vi "DAQ - close all tasks.vi"(8 "Frame Rate":refnum<k21>, 9 "Camera Gate":refnum<k21>, 10 "LED Gate":refnum<k21>, 11 "clock":refnum<k21>) -> (0 "error out":errorcluster)   [LabVIEW 2010]
panel:
  in  "error in":errorcluster
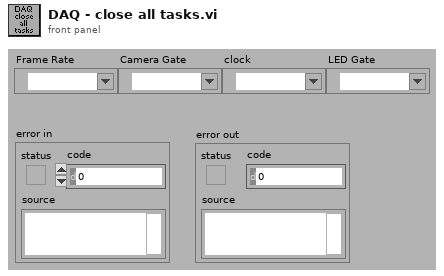
[diagram p1: front panel]
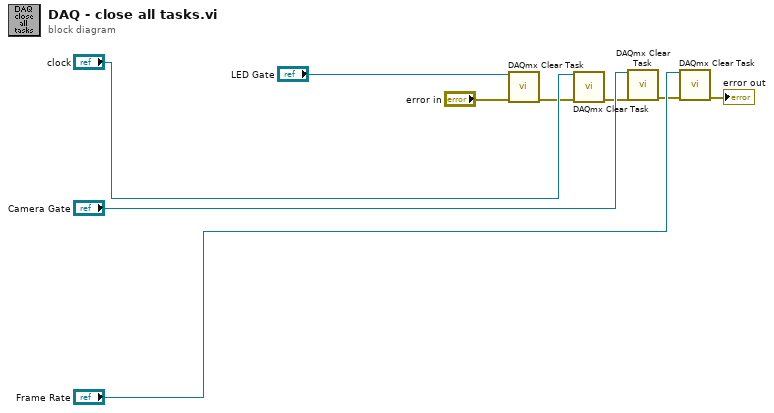
[diagram p0: block diagram]
diagram:
  n1 = call <vilib>:"DAQmx Clear Task.vi"("task in"="LED Gate", "error in"="error in") -> ("error out"=w4:errorcluster)  [unwired: 13 in]
  n2 = call <vilib>:"DAQmx Clear Task.vi"("task in"="clock", "error in"=w4) -> ("error out"=w1:errorcluster)  [unwired: 13 in]
  n3 = call <vilib>:"DAQmx Clear Task.vi"("task in"="Camera Gate", "error in"=w1) -> ("error out"=w2:errorcluster)  [unwired: 13 in]
  n4 = call <vilib>:"DAQmx Clear Task.vi"("task in"="Frame Rate", "error in"=w2) -> ("error out"=→"error out":errorcluster)  [unwired: 13 in]
